vi "Start Action.vi"(8 "error in (no error)":errorcluster, 11 "Device in":refnum<class "Device.lvclass">) -> (0 "error out":errorcluster, 3 "Device out":refnum<class "Device.lvclass">)   [LabVIEW 2023, in "Device.lvlib" / "Device.lvclass"]
uses:
  Device.lvclass
  Device.lvclass/Device.ctl
  <vilib>/ActorFramework/Message Enqueuer/Message Enqueuer.lvclass/Message Enqueuer.ctl
  Device Messages/Perform Action Msg/Perform Action Msg.lvclass
  C:/Program Files (x86)/National Instruments/LabVIEW 2023/vi.lib/ActorFramework/Message/Message.lvclass
  <vilib>/ActorFramework/Message Enqueuer/Enqueue.vi
  <vilib>/ActorFramework/Message Priority Queue/Priority Enqueue.vi
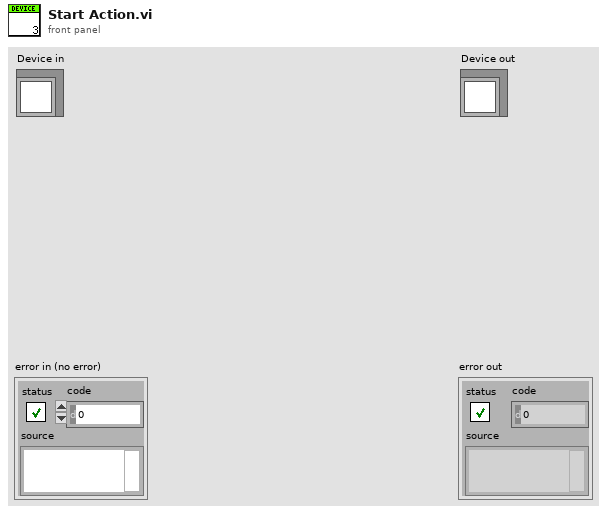
[diagram p1: front panel]
types:
  T1 = typedef "Device.lvlib/Device.lvclass/cyclical pattern.ctl" = enum16{"No Loop", "Fastest", "Timer"}
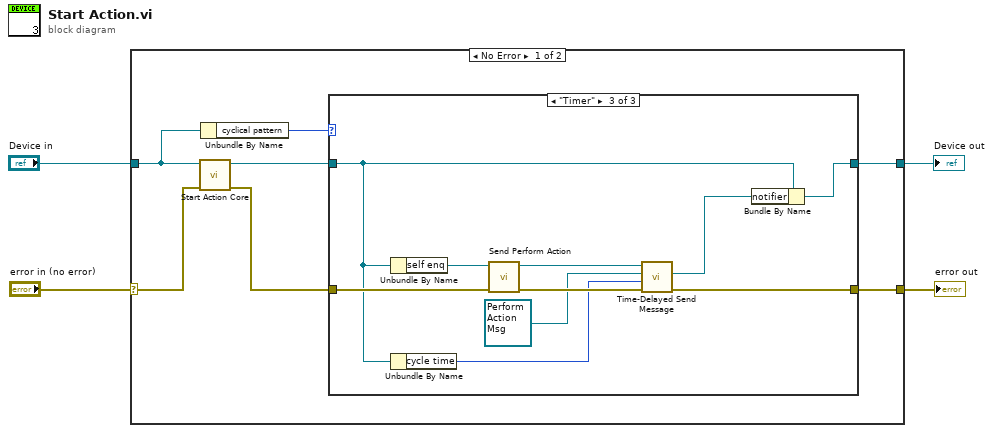
[diagram p0: block diagram]
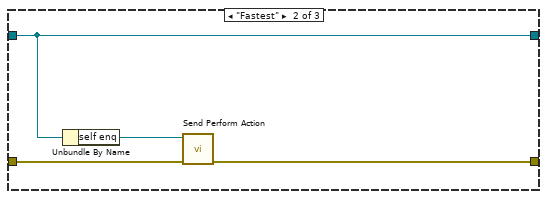
[diagram p3: hidden frame]
diagram:
  n1 = case shown="No Error" "error in (no error)" {
    selector: "error in (no error)" -> [w11 w29]
    tunnel: [w6 w29] -> w3
    tunnel: [w5 w28] -> w1
    tunnel: "Device in" -> [w10 w28]
    frame No Error {
      n2 = call-dynamic "Start Action Core.vi"("error in (no error)"=w11, "Device in"=w10) -> ("error out"=w7:errorcluster, "Device out"=w8:refnum<class "Device.lvclass">)  [unwired: 8 in]
      n3 = Unbundle By Name(w10) -> ("cyclical pattern"=w9:T1)
      n4 = case shown="\"Timer\"" w9 {
        tunnel: w8 -> [w12 w15 w19]
        tunnel: w7 -> [w13 w17 w26]
        tunnel: [w13 w16 w21] -> w6
        tunnel: [w12 w15 w27] -> w5
        frame "No Loop", Default {
        }
        frame "Fastest" {
          n5 = Unbundle By Name(w15) -> ("self enq"=w14:refnum<class "Message Enqueuer.lvclass">)
          n6 = call "Send Perform Action.vi"("error in (no error)"=w17, "Message Enqueuer"=w14) -> ("error out"=w16:errorcluster)  [unwired: 8 in, 1 out]
        }
        frame "Timer" {
          n7 = Unbundle By Name(w19) -> ("self enq"=w18:refnum<class "Message Enqueuer.lvclass">)
          n8 = Unbundle By Name(w19) -> ("cycle time"=w20:u32)
          n9 = call "Send Perform Action.vi"("error in (no error)"=w26, "Message Enqueuer"=w18) -> ("error out"=w25:errorcluster, "Message Enqueuer out"=w24:refnum<class "Message Enqueuer.lvclass">)  [unwired: 8 in]
          n10 = call <vilib>:"Time-Delayed Send Message.vi"("error in (no error)"=w25, "Milliseconds To Wait"=w20, "Message"=refnum<class "Perform Action Msg.lvclass"> refnum ("Perform Action Msg.lvclass"), "Message Enqueuer"=w24) -> ("error out"=w21:errorcluster, "Delivery Notifier"=w22:refnum<notifier>)  [unwired: 6 in]
          n11 = Bundle By Name(cluster=w19, "notifier"=w22) -> (w27:refnum<class "Device.lvclass">)
        }
      }
    }
    frame Error {
    }
  }
  "error out" <- w3
  "Device out" <- w1
